vi "Init Object.vi"(6 "Minimal size [0, 0]":cluster{"Horizontal":i16, "Vertical":i16}, 7 "GObj Refnum":refnum<vi>, 8 "error in (no error)":errorcluster, 9 "B [0, 0, 0, 0]":T1, 10 "A [0, 0, 1, 1]":T1={"Left"=0.0, "Top"=0.0, "Right"=1.0, "Bottom"=1.0}) -> (0 "error out":errorcluster, 3 "MMI Scaling out":refnum<class "Object.lvclass">)   [LabVIEW 2021, in "Object.lvclass"]
uses:
  Object.lvclass
  Object.lvclass/Object.ctl
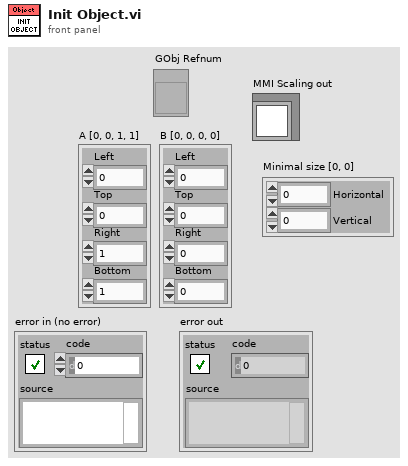
[diagram p1: front panel]
types:
  T1 = cluster{"Left":dbl, "Top":dbl, "Right":dbl, "Bottom":dbl}
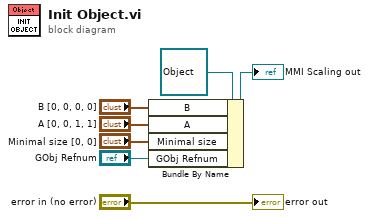
[diagram p0: block diagram]
diagram:
  n1 = Bundle By Name(cluster=refnum<class "Object.lvclass"> refnum ("MMI Scaling in"), "B"="B [0, 0, 0, 0]", "A"="A [0, 0, 1, 1]", "Minimal size"="Minimal size [0, 0]", "GObj Refnum"="GObj Refnum") -> (→"MMI Scaling out":refnum<class "Object.lvclass">)
  "error out" <- "error in (no error)"
